vi "ODBC_Write.vi"(1 "Query":string, 2 "Database File":path) -> (0 "Error":bool)   [LabVIEW 2011]
doc: "This VI executes a given SQL query on a Microsoft Access database."
uses:
  odbc_labview.dll
panel:
  out "error out":errorcluster
  out "result string":string
  out "return type":i32
  out "output string":string
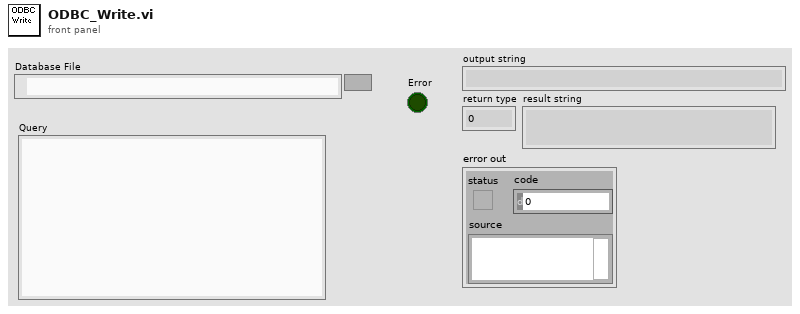
[diagram p1: front panel]
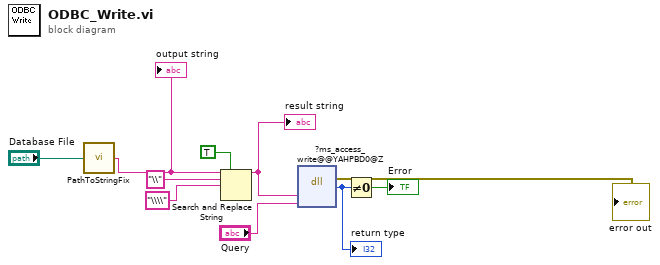
[diagram p0: block diagram]
diagram:
  n1 = call "PathToStringFix.vi"("path 2"="Database File") -> ("output string"=w2:string)
  "output string" <- w2
  n2 = Search and Replace String(replace all?=TRUE ("replace all? (F)"), input string=w2, search string="\\", replace string="\\\\" ("replace string (\"\")")) -> (result string=w7:string)  [unwired: 4 in, 3 out]
  "result string" <- w7
  n3 = dll-call lib="C:/MOCVD/MOCVD_LabView2011/MOCVD_Lib_v14_dev/editor_lib/odbc/odbc_labview.dll" fn="?ms_access_write@@YAHPBD0@Z"("arg1"=w7, "arg2"="Query") -> (error out=→"error out":errorcluster, "return type"=w4:i32)  [unwired: 5 in, 1 out]
  "return type" <- w4
  n4 = Not Equal To 0?(x=w4) -> (x != 0?=→"Error":bool)
